vi "Write GCD Error Log File.vi"(4 "Write File":bool=TRUE, 5 "Write Mode":bool, 6 "Initialize":bool, 7 "Error Out Mode":T1(ring), 8 "Error In":errorcluster, 10 "Test Mode":T2(ring), 11 "Log File Name":string="GCD Error.log") -> (0 "Error Out":errorcluster, 1 "Last Err":bool, 2 "Logged":bool, 3 "LineOut":string)   [LabVIEW 2013]
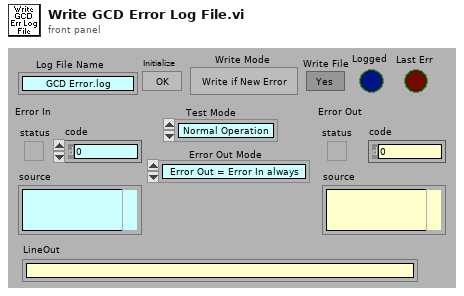
[diagram p1: front panel]
types:
  T1 = enum16{"Error Out = Error In always", "Always Cleared", "Error Out = Error In if Logged"}
  T2 = enum16{"Normal Operation", "Test - No Error", "Test - Error 1", "Test - Error 2"}
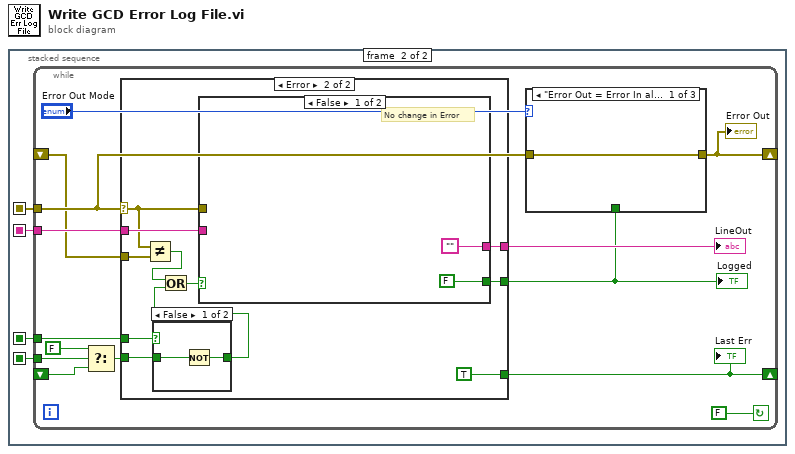
[diagram p0: block diagram]
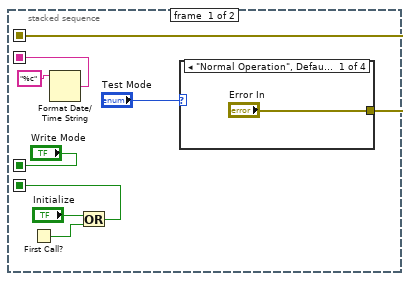
[diagram p2: hidden frame]
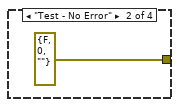
[diagram p3: hidden frame]
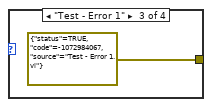
[diagram p4: hidden frame]
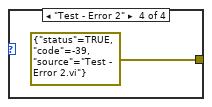
[diagram p5: hidden frame]
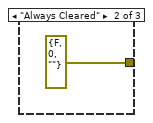
[diagram p6: hidden frame]
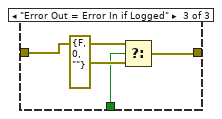
[diagram p7: hidden frame]
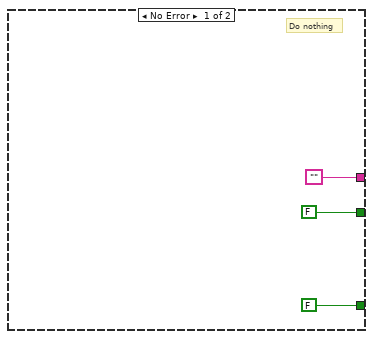
[diagram p8: hidden frame]
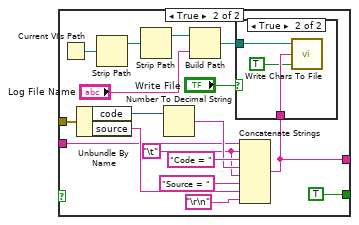
[diagram p9: hidden frame]
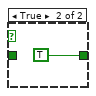
[diagram p11: hidden frame]
diagram:
  n1 = stacked-sequence {
    seq-local: [w6 _] -> [_ w16]
    seq-local: ["Write Mode" _] -> [_ w15]
    seq-local: [w1 _] -> [_ w14]
    seq-local: [w4 _] -> [_ w13]
    frame #0 {
      n2 = First Call?() -> (First Call?: T/F=w3:bool)
      n3 = Format Date/Time String(time format string (%c)="%c") -> (date/time string=w4:string)  [unwired: 2 in]
      n4 = Or(x="Initialize", y=w3) -> (x .or. y?=w1:bool)
      n5 = case shown="\"Normal Operation\", Default" "Test Mode" {
        tunnel: ["Error In" errorcluster {"status"=FALSE, "code"=0, "source"=""} ("Error In") errorcluster {"status"=TRUE, "code"=-1072984067, "source"="Test - Error 1.vi"} ("Error In") errorcluster {"status"=TRUE, "code"=-39, "source"="Test - Error 2.vi"} ("Error In")] -> w6
        frame "Normal Operation", Default {
        }
        frame "Test - No Error" {
        }
        frame "Test - Error 1" {
        }
        frame "Test - Error 2" {
        }
      }
    }
    frame #1 {
      n6 = while {
        tunnel: w16 -> [w20]
        shift-right: [w22] -> _
        shift-left: _ -> [w27]
        tunnel: w15 -> [w29]
        tunnel: w14 -> [w28]
        tunnel: w13 -> [w24]
        shift-right: [w17] -> _
        shift-left: _ -> [w18]
        stop <- FALSE continue-if-true
        n7 = Select(t=FALSE, s=w28, f=w27) -> (s? t:f=w26:bool)
        n8 = case shown="Error" w20 {
          selector: w20 -> [_ w42]
          tunnel: w26 -> [_ w48]
          tunnel: [FALSE TRUE] -> w22
          tunnel: w29 -> [_ w49]
          tunnel: w24 -> [_ w47]
          tunnel: [FALSE w45] -> w19
          tunnel: ["" w44] -> w23
          tunnel: w18 -> [_ w41]
          frame No Error {
            # "Do nothing"
          }
          frame Error {
            n9 = Not Equal?(x=w42, y=w41) -> (x != y?=w40:bool)
            n10 = case shown="False" w49 {
              tunnel: w48 -> [w74 _]
              tunnel: [w73 TRUE] -> w46
              frame False {
                n11 = Not(x=w74) -> (.not. x?=w73:bool)
              }
              frame True {
              }
            }
            n12 = Or(x=w40, y=w46) -> (x .or. y?=w43:bool)
            n13 = case shown="False" w43 {
              tunnel: w42 -> [_ w64]
              tunnel: w47 -> [_ w55]
              tunnel: [FALSE TRUE] -> w45
              tunnel: ["" w53] -> w44
              frame False {
                # "No change in Error"
              }
              frame True {
                w59 = "\t"
                n14 = Current VI's Path() -> (path=w66:path)
                n15 = Unbundle By Name(w64) -> ("code"=w62:i32, "source"=w56:string)
                n16 = Strip Path(path=w66) -> (stripped path=w67:path)  [unwired: 1 out]
                n17 = Strip Path(path=w67) -> (stripped path=w68:path)  [unwired: 1 out]
                n18 = Number To Decimal String(number=w62) -> (decimal integer string=w60:string)  [unwired: 1 in]
                n19 = Build Path(base path=w68, name or relative path="Log File Name") -> (appended path=w65:path)
                n20 = Concatenate Strings(w55, w59, "Code = " ("string"), w60, w59, "Source = " ("string"), w56, "\r\n") -> (w53:string)
                n21 = case shown="True" "Write File" {
                  tunnel: w65 -> [_ w72]
                  tunnel: w53 -> [_ w71]
                  frame False {
                  }
                  frame True {
                    n22 = call "Write Chars To File.vi"("append to file? (new file:F)"=TRUE, "character string"=w71, "file path (dialog if empty)"=w72) -> ()  [unwired: 2 in, 1 out]
                  }
                }
              }
            }
          }
        }
        "Logged" <- w19
        "LineOut" <- w23
        "Last Err" <- w22
        n23 = case shown="\"Error Out = Error In always\", Default" "Error Out Mode" {
          tunnel: [w31 errorcluster {"status"=FALSE, "code"=0, "source"=""} ("Error In") w35] -> w17
          tunnel: w20 -> [w31 _ w34]
          tunnel: w19 -> [_ _ w33]
          frame "Error Out = Error In always", Default {
          }
          frame "Always Cleared" {
          }
          frame "Error Out = Error In if Logged" {
            n24 = Select(t=w34, s=w33, f=errorcluster {"status"=FALSE, "code"=0, "source"=""} ("Error In")) -> (s? t:f=w35:errorcluster)
          }
        }
        "Error Out" <- w17
      }
    }
  }
